vi "defendGoalTacticCheckStateChange.vi"(8 "error in (no error)":errorcluster, 9 "Robot In":refnum<class "Robot.lvclass">, 10 "Game in":refnum<class "Game.lvclass">, 11 "DefendGoalTacticVSS in":refnum<class "DefendGoalTacticVSS.lvclass">) -> (0 "error out":errorcluster, 2 "States":T1=enum."DefBallPos", 3 "DefendGoalTacticVSS out":refnum<class "DefendGoalTacticVSS.lvclass">)   [LabVIEW 2023, in "DefendGoalTacticVSS.lvclass"]
uses:
  DefendGoalTacticVSS.lvclass
  Game_class/Game.lvclass
  Robot_class/Robot.lvclass
  C:/Users/ivoli/OneDrive/Documentos/GitHub/VSS_AI/Object_class/Object.lvclass
  DefendGoalStates.ctl
  Utilities_class/Utilities.lvclass
  Game_class/Game.lvclass/Game.ctl
  Game_class/Read BallRef.vi
  Object_class/Read x.vi
  Ball_class/Ball.lvclass
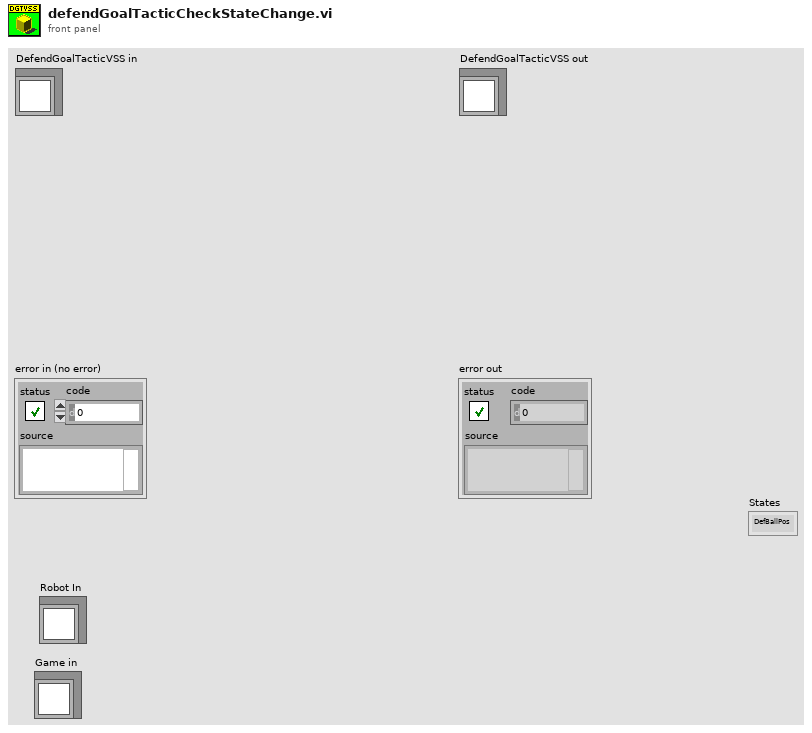
[diagram p1: front panel]
types:
  T1 = typedef "DefendGoalStates.ctl" = enum16{"Kick", "DefBallPos", "SpillSkin", "Exit"}
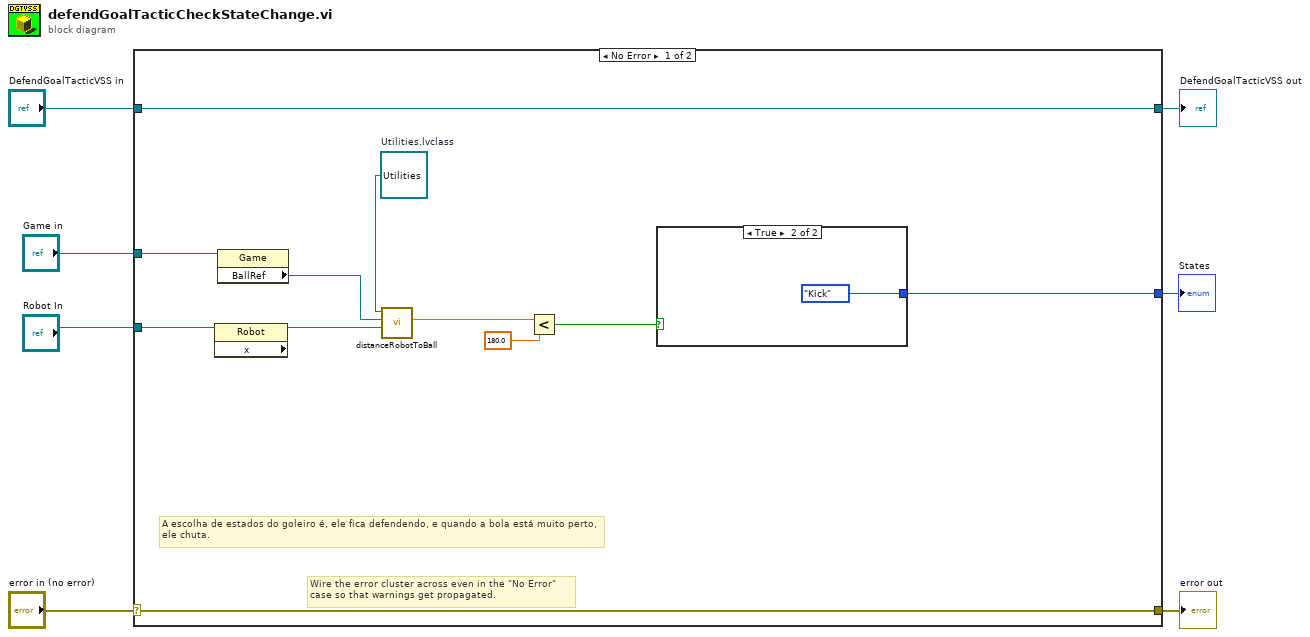
[diagram p0: block diagram]
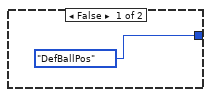
[diagram p2: hidden frame]
diagram:
  n1 = case shown="No Error" "error in (no error)" {
    selector: "error in (no error)" -> [w17 w22]
    tunnel: [w17 w22] -> w6
    tunnel: [w18 w21] -> w4
    tunnel: "DefendGoalTacticVSS in" -> [w18 w21]
    tunnel: [w16 _] -> w1
    tunnel: "Robot In" -> [w15 _]
    tunnel: "Game in" -> [w14 _]
    frame No Error {
      w12 = refnum<class "Utilities.lvclass"> refnum  # Utilities.lvclass
      # "A escolha de estados do goleiro é, ele fica defendendo, e quando a bola está muito perto, ele chuta."
      # "Wire the error cluster across even in the \"No Error\"\ncase so that warnings get propagated."
      n2 = property class="Robot" props=["x"](reference=w15) -> (reference out=w11:refnum<class "Robot.lvclass">)  [unwired: 1 in, 2 out]
      n3 = property class="Game"(reference=w14) -> ("BallRef"=w9:refnum<class "Ball.lvclass">)  [unwired: 1 in, 2 out]
      n4 = call "distanceRobotToBall.vi"("Robot"=w11, "Ball"=w9, "Utilities in"=w12) -> ("Distance Robot To Ball"=w10:dbl)  [unwired: 6 in, 2 out]
      n5 = Less?(x=w10, y=180.0) -> (x < y?=w8:bool)
      n6 = case shown="True" w8 {
        tunnel: [DefendGoalStates."DefBallPos" ("States") DefendGoalStates."Kick" ("States")] -> w16
        frame False {
        }
        frame True {
        }
      }
    }
    frame Error {
    }
  }
  "error out" <- w6
  "DefendGoalTacticVSS out" <- w4
  "States" <- w1
